vi "Save as JUnit.vi"(8 "Error In (No Error)":errorcluster, 10 "Analysis Results":T9 {"Test Config Data"."Test Ranking" items=["Low", "Normal", "High"]}, 11 "XML file path":path) -> (0 "Error Out":errorcluster)   [LabVIEW 2014, in "VI Analyzer Parsing.lvlib"]
uses:
  VI Analyzer Parsing.lvlib
  <vilib>/addons/analyzer/_analyzerctrls.llb/VIAnCtl Results.ctl
  <vilib>/addons/analyzer/_analyzerctrls.llb/VIAnCtl ResultsData (index).ctl
  <vilib>/addons/analyzer/_analyzerctrls.llb/VIAnCtl ResultStatus.ctl
  <vilib>/addons/analyzer/_vianresshared.llb/VIAnRes Parsed Results Data (by VI).ctl
  <vilib>/addons/analyzer/_vianresshared.llb/VIAnRes Parsed Results Data (by Test).ctl
  <vilib>/addons/analyzer/_analyzerctrls.llb/VIAnCtl Test Config Data.ctl
  <vilib>/addons/analyzer/_analyzerctrls.llb/VIAnCtl TestRanking.ctl
  <vilib>/addons/analyzer/_analyzerctrls.llb/VIAnCtl Config Control Value.ctl
  <vilib>/NI/JUnit Results API/Controls/Test Suite Attribute Values.ctl
  <vilib>/xml/Close Reference(Node).vi
  <vilib>/xml/NI_XML.lvlib
  <vilib>/NI/JUnit Results API/JUnit API.lvlib
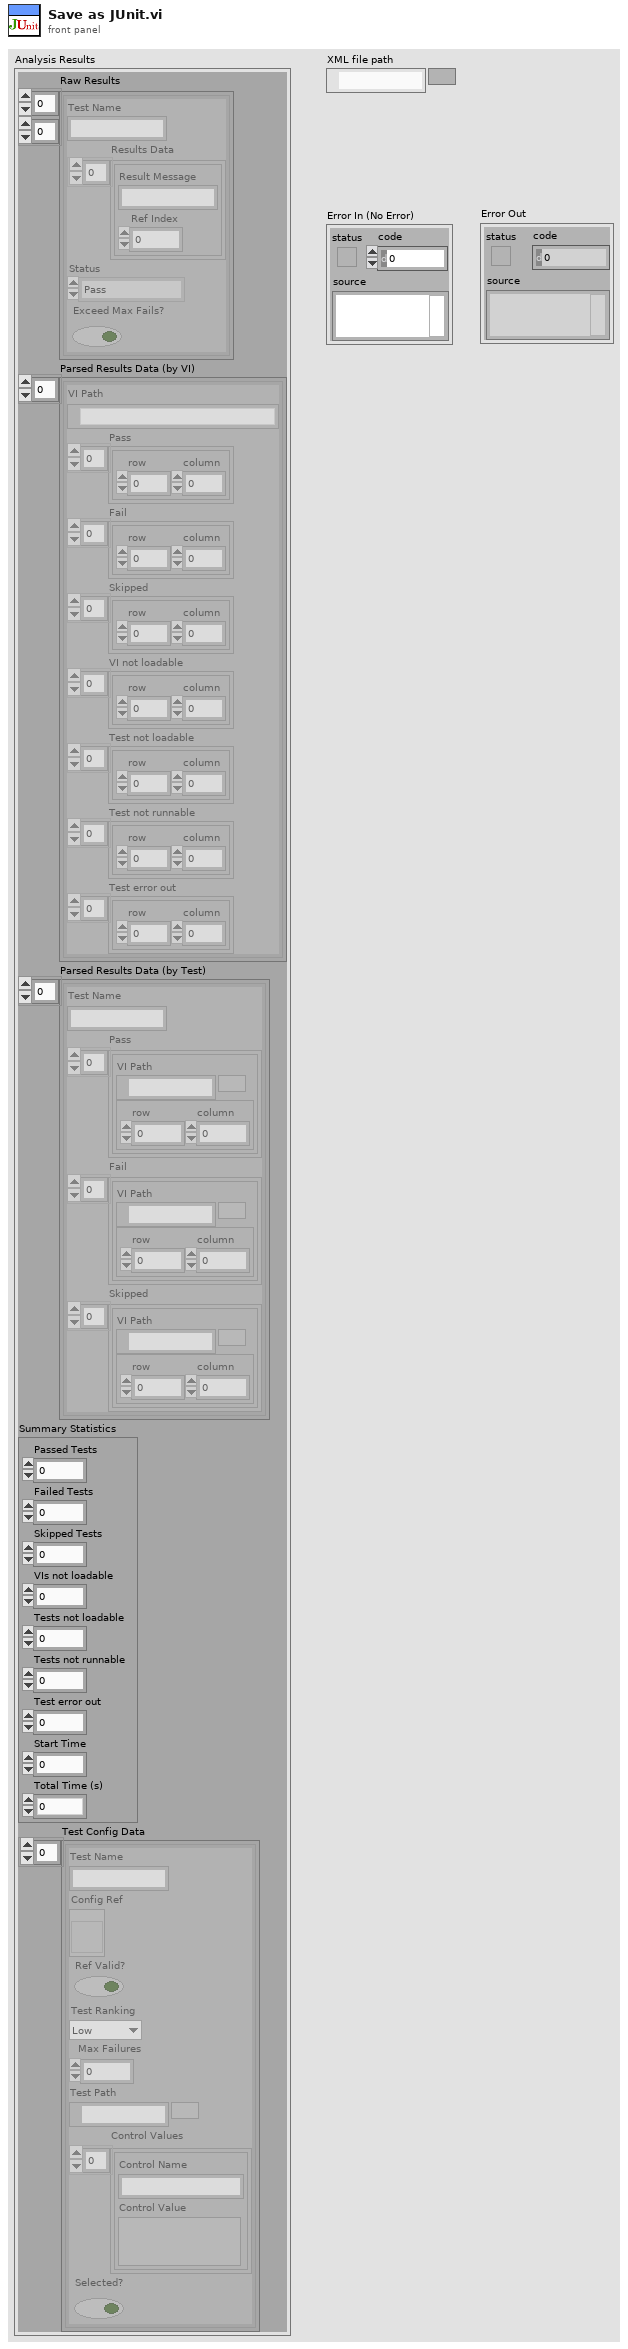
[diagram p1: front panel]
types:
  T1 = typedef "VIAnCtl Results.ctl" = cluster{"Test Name":string, "Results Data":T2[], "Status":T3, "Exceed Max Fails?":bool}
  T2 = typedef "VIAnCtl ResultsData (index).ctl" = cluster{"Result Message":string, "Ref Index":i32}
  T3 = typedef "VIAnCtl ResultStatus.ctl" = enum16{"Pass", "Fail", "Skipped", "VI not loadable", "Test not loadable", "Test not runnable", "Test error out"}
  T4 = typedef "VIAnRes Parsed Results Data (by VI).ctl" = cluster{"VI Path":path, "Pass":cluster{"row":i32, "column":i32}[], "Fail":cluster{"row":i32, "column":i32}[], "Skipped":cluster{"row":i32, "column":i32}[], "VI not loadable":cluster{"row":i32, "column":i32}[], "Test not loadable":cluster{"row":i32, "column":i32}[], "Test not runnable":cluster{"row":i32, "column":i32}[], "Test error out":cluster{"row":i32, "column":i32}[]}
  T5 = typedef "VIAnRes Parsed Results Data (by Test).ctl" = cluster{"Test Name":string, "Pass":cluster{"VI Path":path, "index":cluster{"row":i32, "column":i32}}[], "Fail":cluster{"VI Path":path, "index":cluster{"row":i32, "column":i32}}[], "Skipped":cluster{"VI Path":path, "index":cluster{"row":i32, "column":i32}}[]}
  T6 = typedef "VIAnCtl Test Config Data.ctl" = cluster{"Test Name":string, "Config Ref":refnum<vi>, "Ref Valid?":bool, "Test Ranking":T7, "Max Failures":u32, "Test Path":path, "Control Values":T8[], "Selected?":bool}
  T7 = typedef "VIAnCtl TestRanking.ctl" = u16
  T8 = typedef "VIAnCtl Config Control Value.ctl" = cluster{"Control Name":string, "Control Value":variant}
  T9 = cluster{"Raw Results":T1[][], "Parsed Results Data (by VI)":T4[], "Parsed Results Data (by Test)":T5[], "Summary Statistics":cluster{"Passed Tests":i32, "Failed Tests":i32, "Skipped Tests":i32, "VIs not loadable":i32, "Tests not loadable":i32, "Tests not runnable":i32, "Test error out":i32, "Start Time":u32, "Total Time (s)":dbl}, "Test Config Data":T6[]}
  T10 = typedef "JUnit API.lvlib/Test Suite Attribute Values.ctl" = cluster{"name":string, "tests":i32, "failures":i32, "errors":i32, "time":dbl, "disabled":i32, "skipped":i32, "skips":i32, "timestamp":dbl, "hostname":string, "id":string, "package":string, "assertions":i32, "file":string, "skip":string, "log":string, "url":string}
  T11 = cluster{"Pass":cluster{"row":i32, "column":i32}[]}
  T12 = cluster{"Fail":cluster{"row":i32, "column":i32}[]}
  T13 = cluster{"Skipped":cluster{"row":i32, "column":i32}[]}
  T14 = cluster{"VI not loadable":cluster{"row":i32, "column":i32}[]}
  T15 = cluster{"Test not loadable":cluster{"row":i32, "column":i32}[]}
  T16 = cluster{"Test not runnable":cluster{"row":i32, "column":i32}[]}
  T17 = cluster{"Test error out":cluster{"row":i32, "column":i32}[]}
  T18 = cluster{"Test error out":cluster{"row":i32, "column":i32}[]}[]
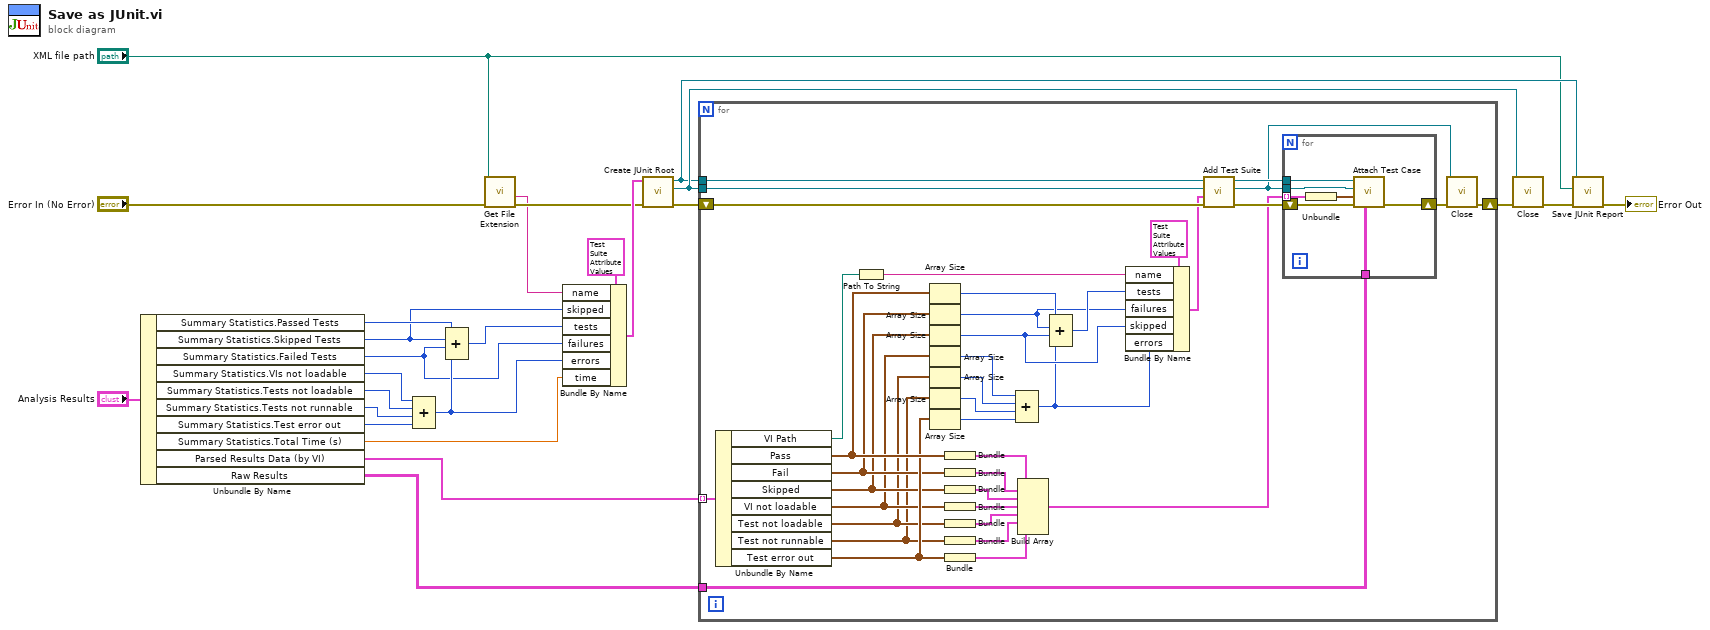
[diagram p0: block diagram]
diagram:
  n1 = Unbundle By Name("Analysis Results") -> ("Summary Statistics.Passed Tests"=w9:i32, "Summary Statistics.Skipped Tests"=w1:i32, "Summary Statistics.Failed Tests"=w2:i32, "Summary Statistics.VIs not loadable"=w8:i32, "Summary Statistics.Tests not loadable"=w7:i32, "Summary Statistics.Tests not runnable"=w6:i32, "Summary Statistics.Test error out"=w5:i32, "Summary Statistics.Total Time (s)"=w4:dbl, "Parsed Results Data (by VI)"=w19:T4[], "Raw Results"=w18:T1[][])
  n2 = Compound Arithmetic op=ADD(w8, w7, w6, w5) -> (w3:i32)
  n3 = Compound Arithmetic op=ADD(w9, w1, w2, w3) -> (w20:i32)
  n4 = call <vilib>:"Get File Extension.vi"("error in (no error)"="Error In (No Error)", "file"="XML file path") -> ("error out"=w11:errorcluster, "filename without extension"=w10:string)  [unwired: 6 in, 2 out]
  n5 = Bundle By Name(cluster=T10 {"name"="", "tests"=-1, "failures"=-1, "errors"=-1, "time"=-1.0, "disabled"=-1, "skipped"=-1, "skips"=-1, "timestamp"=-1.0, "hostname"="", "id"="", "package"="", "assertions"=-1, "file"="", "skip"="", "log"="", "url"=""} ("Test Suites Atrributes"), "name"=w10, "skipped"=w1, "tests"=w20, "failures"=w2, "errors"=w3, "time"=w4) -> (w23:T10)
  n6 = call <vilib>:"Create JUnit Root.vi"("Error In (No Error)"=w11, "Test Suites Atrributes"=w23) -> ("Error Out"=w24:errorcluster, "Teststuites Ref"=w15:refnum<k20>, "File Ref Out"=w14:refnum<k20>)  [unwired: 7 in]
  n7 = for {
    tunnel: w15 -> [w60]
    shift-right: [w30] -> w17
    shift-left: w24 -> [w63]
    tunnel: w19 -> [w55] mode=indexing
    tunnel: w18 -> [w46]
    tunnel: w14 -> [w61]
    n8 = Unbundle By Name(w55) -> ("VI Path"=w53:path, "Pass"=w45:cluster{"row":i32, "column":i32}[], "Fail"=w43:cluster{"row":i32, "column":i32}[], "Skipped"=w42:cluster{"row":i32, "column":i32}[], "VI not loadable"=w41:cluster{"row":i32, "column":i32}[], "Test not loadable"=w40:cluster{"row":i32, "column":i32}[], "Test not runnable"=w39:cluster{"row":i32, "column":i32}[], "Test error out"=w44:cluster{"row":i32, "column":i32}[])
    n9 = Path To String(path=w53) -> (string=w54:string)
    n10 = Array Size(array=w45) -> (size(s)=w49:i32)
    n11 = Array Size(array=w43) -> (size(s)=w28:i32)
    n12 = Array Size(array=w42) -> (size(s)=w27:i32)
    n13 = Array Size(array=w41) -> (size(s)=w48:i32)
    n14 = Array Size(array=w40) -> (size(s)=w50:i32)
    n15 = Array Size(array=w39) -> (size(s)=w51:i32)
    n16 = Array Size(array=w44) -> (size(s)=w52:i32)
    n17 = Bundle("Pass"=w45) -> (w38:T11)  [unwired: 1 in]
    n18 = Bundle("Fail"=w43) -> (w35:T12)  [unwired: 1 in]
    n19 = Bundle("Skipped"=w42) -> (w34:T13)  [unwired: 1 in]
    n20 = Bundle("VI not loadable"=w41) -> (w36:T14)  [unwired: 1 in]
    n21 = Bundle("Test not loadable"=w40) -> (w32:T15)  [unwired: 1 in]
    n22 = Bundle("Test not runnable"=w39) -> (w33:T16)  [unwired: 1 in]
    n23 = Bundle("Test error out"=w44) -> (w37:T17)  [unwired: 1 in]
    n24 = Compound Arithmetic op=ADD(w48, w50, w51, w52) -> (w26:i32)
    n25 = Build Array(w38, w35, w34, w36, w32, w33, w37) -> (w31:T18)
    n26 = Compound Arithmetic op=ADD(w49, w28, w27, w26) -> (w47:i32)
    n27 = Bundle By Name(cluster=T10 {"name"="", "tests"=-1, "failures"=-1, "errors"=-1, "time"=-1.0, "disabled"=-1, "skipped"=-1, "skips"=-1, "timestamp"=-1.0, "hostname"="", "id"="", "package"="", "assertions"=-1, "file"="", "skip"="", "log"="", "url"=""} ("Test Suites Atrributes"), "name"=w54, "tests"=w47, "failures"=w28, "skipped"=w27, "errors"=w26) -> (w56:T10)
    n28 = call <vilib>:"Add Test Suite.vi"("Error In (No Error)"=w63, "Test Suite Atrributes"=w56, "Teststuites Ref In"=w60, "File Ref In"=w61) -> ("Error Out"=w62:errorcluster, "Testsuite Ref"=w29:refnum<k20>, "File Ref Out"=w59:refnum<k20>)  [unwired: 4 in, 1 out]
    n29 = for {
      tunnel: w46 -> [w66]
      shift-right: [w67] -> w58
      shift-left: w62 -> [w70]
      tunnel: w31 -> [w65] mode=indexing
      tunnel: w59 -> [w68]
      tunnel: w29 -> [w69]
      n30 = Unbundle(w65) -> ("Test error out"=w64:cluster{"row":i32, "column":i32}[])
      n31 = call "Attach Test Case.vi"("Raw Results"=w66, "error in (no error)"=w70, "Result Indicies"=w64, "Testsuite Ref in"=w69, "File Ref in"=w68) -> ("error out"=w67:errorcluster)  [unwired: 4 in, 2 out]
    }
    n32 = call-poly <vilib>:"Close.vi"("error in (no error)"=w58, "node"=w29) -> ("error out"=w30:errorcluster)  [unwired: 7 in]
  }
  n33 = call-poly <vilib>:"Close.vi"("error in (no error)"=w17, "node"=w15) -> ("error out"=w16:errorcluster)  [unwired: 7 in]
  n34 = call <vilib>:"Save JUnit Report.vi"("Error In (No Error)"=w16, "XML file path"="XML file path", "File Ref In"=w14) -> ("Error Out"=→"Error Out":errorcluster)  [unwired: 8 in]
